vi "ESP call forget acquire.vi"(8 "error in (no error)":errorcluster, 11 "ESP301.lvclass":refnum<class "ESP301.lvclass">) -> (0 "error out":errorcluster, 2 "ESP301 Acq Data":T1, 3 "ESP301.lvclass":refnum<class "ESP301.lvclass">)   [LabVIEW 2020, in "ESP301.lvclass"]
uses:
  ESP301.lvclass
  AcquireTypeDef.ctl
  stop FGV control.ctl
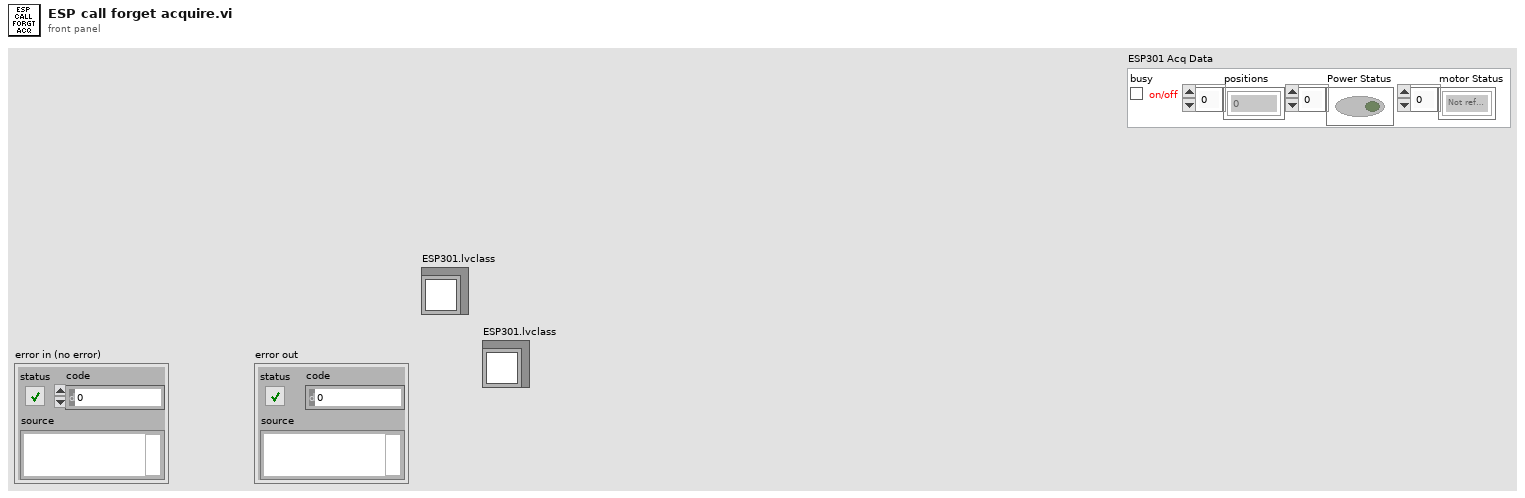
[diagram p1: front panel]
types:
  T1 = typedef "AcquireTypeDef.ctl" = cluster{"busy":bool, "positions":dbl[], "Power Status":bool[], "motor Status":enum16{"Not referenced", "Homing", "Moving", "Ready"}[]}
  T2 = typedef "stop FGV control.ctl" = enum16{"Clear", "Write", "Read"}
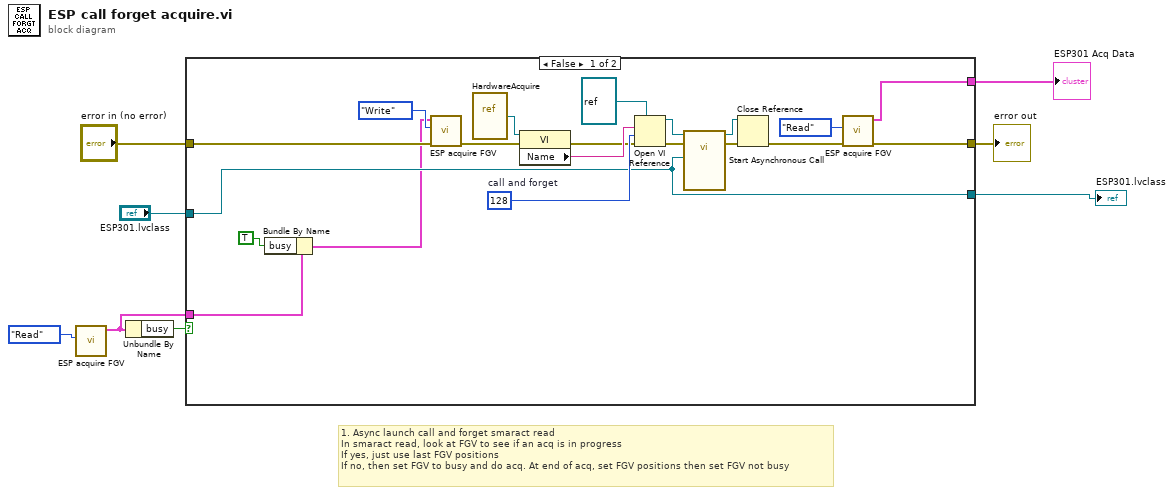
[diagram p0: block diagram]
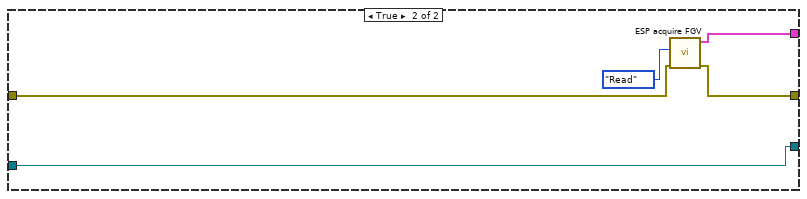
[diagram p2: hidden frame]
diagram:
  # "1. Async launch call and forget smaract read\nIn smaract read, look at FGV to see if an acq is in progress\nIf yes, just use last FGV positions\nIf no, then set FGV to busy and do acq. At end of acq, set FGV positions then set FGV not busy"
  n1 = call "ESP acquire FGV.vi"("Function"=stop_FGV_control."Read") -> ("ESP301 Acq Data"=w4:T1)  [unwired: 9 in, 1 out]
  n2 = Unbundle By Name(w4) -> ("busy"=w6:bool)
  n3 = case shown="False" w6 {
    tunnel: [w14 w33] -> w2
    tunnel: [w11 w29] -> w8
    tunnel: "ESP301.lvclass" -> [w14 w33]
    tunnel: "error in (no error)" -> [w16 w31]
    tunnel: w4 -> [w18 _]
    tunnel: [w9 w30] -> w1
    frame False {
      w28 = 128  # call and forget
      n4 = Bundle By Name(cluster=w18, "busy"=TRUE) -> (w10:T1)
      n5 = call "ESP acquire FGV.vi"("error in"=w16, "Function"=stop_FGV_control."Write", "ESP301 Acq Data"=w10) -> ("error out"=w15:errorcluster)  [unwired: 7 in, 1 out]
      n6 = vi-ref "HardwareAcquire.vi"() -> (w20:refnum<vi>)
      n7 = property class="VI"(reference=w20, error in=w15) -> (error out=w21:errorcluster, "Name"=w22:string)  [unwired: 1 out]
      n8 = Open VI Reference(type specifier VI Refnum (for type only)=refnum<vi> refnum, vi path=w22, options=w28, error in (no error)=w21) -> (vi reference=w26:refnum<vi>, error out=w25:errorcluster)  [unwired: 2 in]
      n9 = call-by-ref "Start Asynchronous Call"(reference=w26, error in=w25, "ESP301 in"=w14) -> (reference out=w23:refnum<vi>, error out=w24:errorcluster)  [unwired: 6 in, 5 out]
      n10 = Close Reference(reference=w23, error in (no error)=w24) -> (error out=w12:errorcluster)
      n11 = call "ESP acquire FGV.vi"("error in"=w12, "Function"=stop_FGV_control."Read") -> ("error out"=w11:errorcluster, "ESP301 Acq Data"=w9:T1)  [unwired: 8 in]
    }
    frame True {
      n12 = call "ESP acquire FGV.vi"("error in"=w31, "Function"=stop_FGV_control."Read") -> ("error out"=w29:errorcluster, "ESP301 Acq Data"=w30:T1)  [unwired: 8 in]
    }
  }
  "error out" <- w8
  "ESP301.lvclass" <- w2
  "ESP301 Acq Data" <- w1
